vi "fit_focus_gauss.vi"(8 "error in":errorcluster, 11 "Focus Measurements":cluster{"focus value":dbl, "height":dbl}[](array[cluster])) -> (0 "error out":errorcluster, 2 "error":dbl, 3 "focus height":dbl)   [LabVIEW 2023, in "Vision.lvlib"]
uses:
  Vision.lvlib
  <vilib>/Analysis/NI_AALPro.lvlib
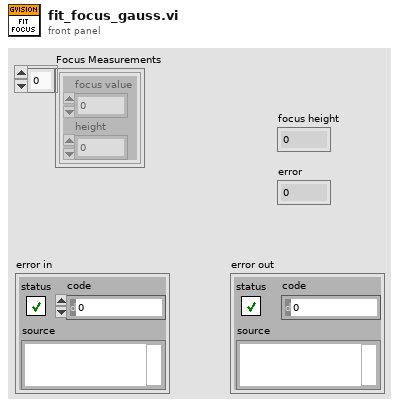
[diagram p1: front panel]
types:
  T1 = cluster{"amp min":dbl, "amp max":dbl, "center min":dbl, "center max":dbl, "deviation min":dbl, "deviation max":dbl, "offset min":dbl, "offset max":dbl}
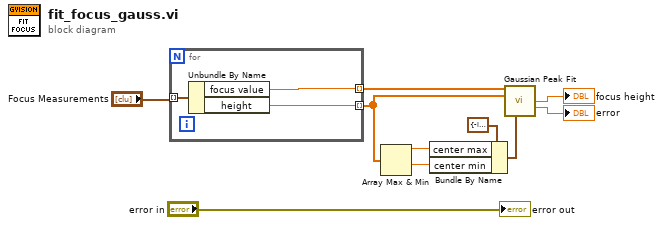
[diagram p0: block diagram]
diagram:
  n1 = for {
    tunnel: "Focus Measurements" -> [w13] mode=indexing
    tunnel: [w11] -> w9 mode=indexing
    tunnel: [w12] -> w1 mode=indexing
    n2 = Unbundle By Name(w13) -> ("focus value"=w11:dbl, "height"=w12:dbl)
  }
  n3 = Array Max & Min(array=w1) -> (max value=w4:dbl, min value=w3:dbl)  [unwired: 2 out]
  n4 = Bundle By Name(cluster=T1 {"amp min"=-inf, "amp max"=inf, "center min"=-inf, "center max"=inf, "deviation min"=-inf, "deviation max"=inf, "offset min"=0.0, "offset max"=0.0} ("parameter bounds"), "center max"=w4, "center min"=w3) -> (w2:T1)
  n5 = call <vilib>:"Gaussian Peak Fit.vi"("Y"=w9, "X"=w1, "parameter bounds"=w2) -> ("center"=→"focus height":dbl, "standard deviation"=→"error":dbl)  [unwired: 6 in, 5 out]
  "error out" <- "error in"
